vi "Publish Group.vi"(8 "error in (no error)":errorcluster, 10 "Group":refnum<class "Group.lvclass">, 11 "VolatusAPI in":refnum<class "VolatusAPI.lvclass">) -> (0 "error out":errorcluster, 3 "VolatusAPI out":refnum<class "VolatusAPI.lvclass">)   [LabVIEW 2020, in "Volatus.lvlib" / "VolatusAPI.lvclass"]
uses:
  VolatusAPI.lvclass
  lv-vecto/Vecto/Group/Group.lvclass
  VolatusAPI.lvclass/VolatusAPI.ctl
  lv-vecto/Vecto/Group/Group.lvclass/Group.ctl
  lv-vecto/Vecto/Group Config/Get Info.vi
  lv-vecto/Vecto/RemoteDataService/RemoteDataService.lvclass
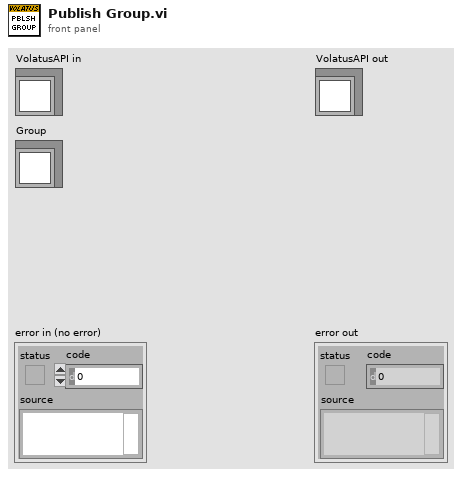
[diagram p1: front panel]
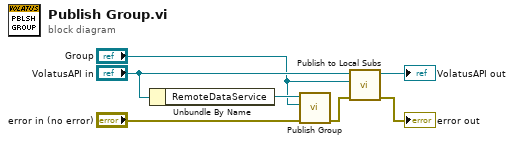
[diagram p0: block diagram]
diagram:
  n1 = Unbundle By Name("VolatusAPI in") -> ("RemoteDataService"=w4:refnum<class "RemoteDataService.lvclass">)
  n2 = call "Publish Group.vi"("error in (no error)"="error in (no error)", "Group"="Group", "RemoteDataService in"=w4) -> ("error out"=w1:errorcluster)  [unwired: 7 in, 1 out]
  n3 = call "Publish to Local Subs.vi"("error in (no error)"=w1, "Group"="Group", "VolatusAPI in"="VolatusAPI in") -> ("error out"=→"error out":errorcluster, "VolatusAPI out"=→"VolatusAPI out":refnum<class "VolatusAPI.lvclass">)  [unwired: 7 in]
